vi "Read ACNET Devices from File.vi"(8 "error in (no error)":errorcluster, 10 "XML File Path":path, 11 "ACNET Devices in":refnum<class "ACNET Devices.lvclass">) -> (0 "error out":errorcluster, 2 "XML File Path (duplicate)":path, 3 "ACNET Devices out":refnum<class "ACNET Devices.lvclass">)   [LabVIEW 2013, in "ACNET Monitor.lvlib"]
uses:
  ACNET Devices.lvclass
  <vilib>/Utility/xml.llb/Read From XML File(string).vi
  ACNET Monitor.lvlib
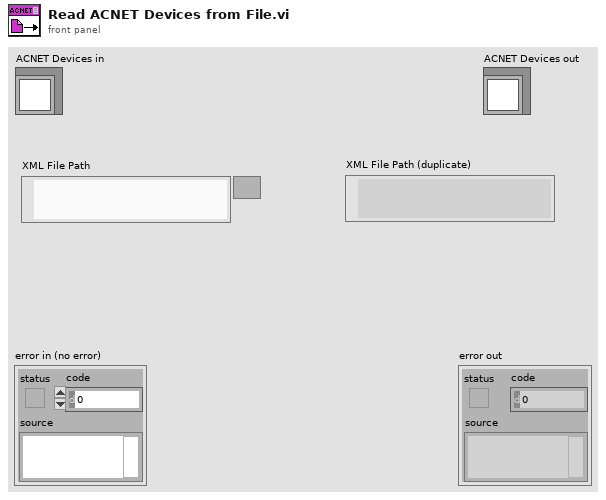
[diagram p1: front panel]
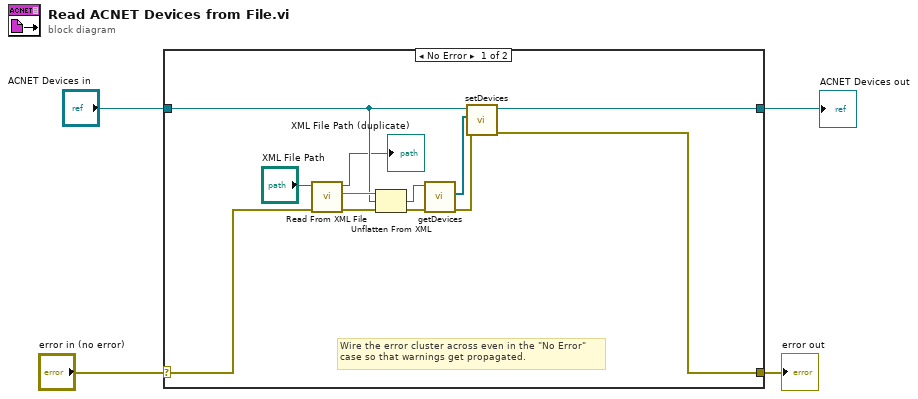
[diagram p0: block diagram]
diagram:
  n1 = case shown="No Error" "error in (no error)" {
    selector: "error in (no error)" -> [w15 w18]
    tunnel: [w7 w18] -> w3
    tunnel: [w8 w17] -> w1
    tunnel: "ACNET Devices in" -> [w10 w17]
    frame No Error {
      # "Wire the error cluster across even in the \"No Error\"\ncase so that warnings get propagated."
      n2 = call-poly <vilib>:"Read From XML File.vi"("error in (no error)"=w15, "XML File Path"="XML File Path") -> ("error out"=w14:errorcluster, "XML Elements"=w13:string, "XML File Path(duplicate)"=→"XML File Path (duplicate)":path)  [unwired: 7 in]
      n3 = Unflatten From XML(xml string=w13, type=w10, error in (no error)=w14) -> (value=w11:refnum<class "ACNET Devices.lvclass">, error out=w12:errorcluster)
      n4 = call-dynamic "getDevices.vi"("error in (no error)"=w12, "ACNET Devices in"=w11) -> ("error out"=w9:errorcluster, "Devices"=w6:refnum<class "ACNET Device.lvclass">[])  [unwired: 7 in, 1 out]
      n5 = call-dynamic "setDevices.vi"("error in (no error)"=w9, "Devices"=w6, "ACNET Devices in"=w10) -> ("error out"=w7:errorcluster, "ACNET Devices out"=w8:refnum<class "ACNET Devices.lvclass">)  [unwired: 7 in]
    }
    frame Error {
    }
  }
  "error out" <- w3
  "ACNET Devices out" <- w1
